vi "Write termChar.vi"(8 "error in (no error)":errorcluster, 10 "termChar":string, 11 "ElectrometerConfiguration in":refnum<class "ElectrometerCOMConfiguration.lvclass">) -> (0 "error out":errorcluster, 3 "ElectrometerConfiguration out":refnum<class "ElectrometerCOMConfiguration.lvclass">)   [LabVIEW 2016, in "ElectrometerCOMConfiguration.lvclass"]
uses:
  ElectrometerCOMConfiguration.lvclass
  ElectrometerCOMConfiguration.lvclass/ElectrometerCOMConfiguration.ctl
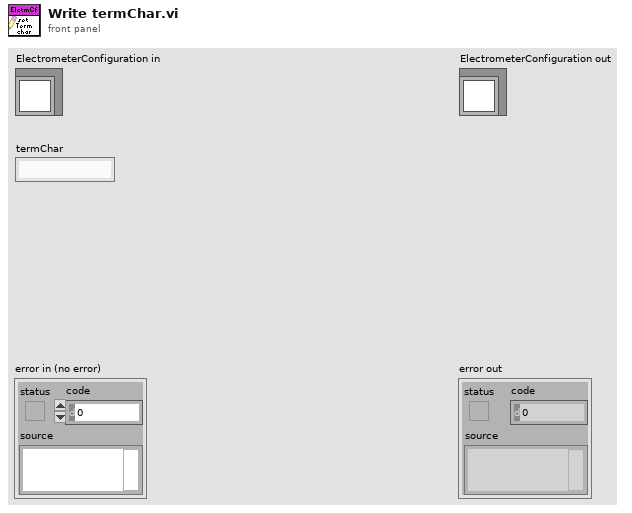
[diagram p1: front panel]
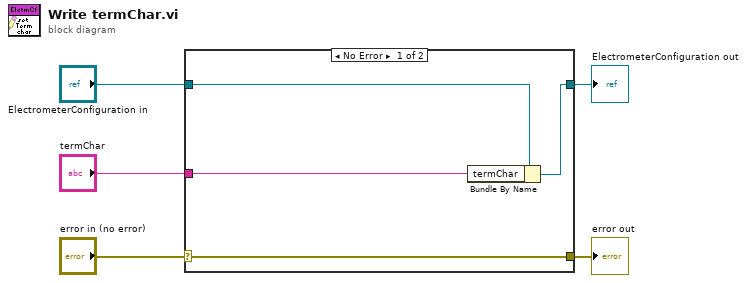
[diagram p0: block diagram]
diagram:
  n1 = case shown="No Error" "error in (no error)" {
    selector: "error in (no error)" -> [w9 w10]
    tunnel: [w9 w10] -> w4
    tunnel: [w7 w11] -> w2
    tunnel: "ElectrometerConfiguration in" -> [w8 w11]
    tunnel: "termChar" -> [w6 _]
    frame No Error {
      n2 = Bundle By Name(cluster=w8, "termChar"=w6) -> (w7:refnum<class "ElectrometerCOMConfiguration.lvclass">)
    }
    frame Error {
    }
  }
  "error out" <- w4
  "ElectrometerConfiguration out" <- w2
